vi "uTransport_IsValid.vi"(8 "error in (no error)":errorcluster, 11 "uClient_Publisher in":refnum<class "uClient_Publisher.lvclass">) -> (0 "error out":errorcluster, 2 "IsValid?":bool, 3 "uClient_Publisher out":refnum<class "uClient_Publisher.lvclass">)   [LabVIEW 2023, in "uLib.lvlib" / "uClient_Publisher.lvclass"]
uses:
  uClient_Publisher.lvclass
  U:/Projects/uLib/Src/uFramework/uClient/uClient.lvclass
  uClient/uClient.lvclass/uClient.ctl
  uClient/uClient_GetTransport.vi
  uTransport/uTransport/uTransport.lvclass
  uClient_Publisher.lvclass/uClient_Publisher.ctl
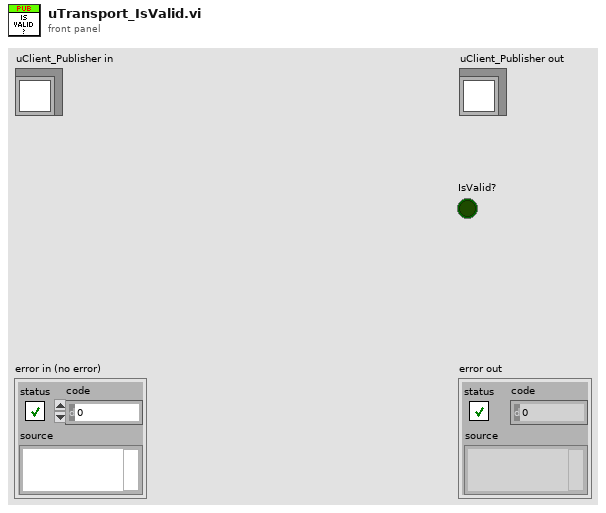
[diagram p1: front panel]
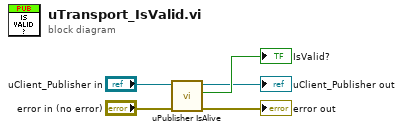
[diagram p0: block diagram]
diagram:
  n1 = call "uPublisher IsAlive.vi"("error in (no error)"="error in (no error)", "uClient_Publisher in"="uClient_Publisher in") -> ("error out"=→"error out":errorcluster, "Is Alive?"=→"IsValid?":bool, "uClient_Publisher out"=→"uClient_Publisher out":refnum<class "uClient_Publisher.lvclass">)  [unwired: 7 in]
